vi "DBL.vi"(4 "Value":T1) -> (1 "Constant":refnum<class "Const_DBL_1D.lvclass">)   [LabVIEW 2021, in "Const_DBL_1D.lvclass"]
uses:
  Const_DBL_1D.lvclass
  Type.ctl
  Const_DBL_1D.lvclass/Const_DBL_1D.ctl
  Properties/Write Value.vi
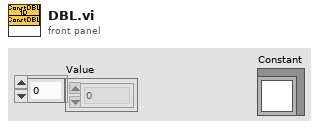
[diagram p1: front panel]
types:
  T1 = typedef "Const_DBL_1D.lvclass/Type.ctl" = dbl[]
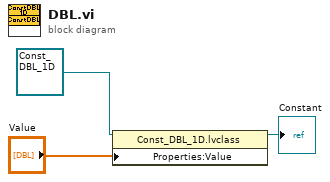
[diagram p0: block diagram]
diagram:
  n1 = property class="Const_DBL_1D.lvclass"(reference=refnum<class "Const_DBL_1D.lvclass"> refnum ("Constants.lvlib:Numeric.lvclass"), "Properties:Value"="Value") -> (reference out=→"Constant":refnum<class "Const_DBL_1D.lvclass">)  [unwired: 1 in, 1 out]
